vi "SampleClient.vi"() -> ()   [LabVIEW 2012]
doc: "A sample client that can be run on the computer or RIO"
panel:
  in  "Service call":bool
  out "Answer":string
  out "ms/iteration":dbl
  in  "Show Web":bool
  in  "LED":bool
  out "time":string
  out "Status":string
  in  "stop":bool
  # "Instructions:\n1. Run the VI\n2. Verify that you see the correct time.\n3. Press the LED button. You should see the LED reply change.\nIf you are targetting a myRIO, the LED should change as well.\n4. Debug by clicking Show Webpage.\n5. See what is being sent back and forth by clicking Show Webpage."
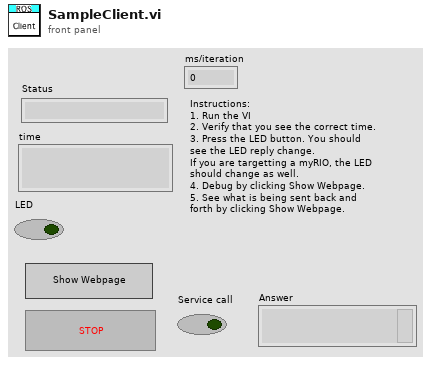
[diagram p1: front panel]
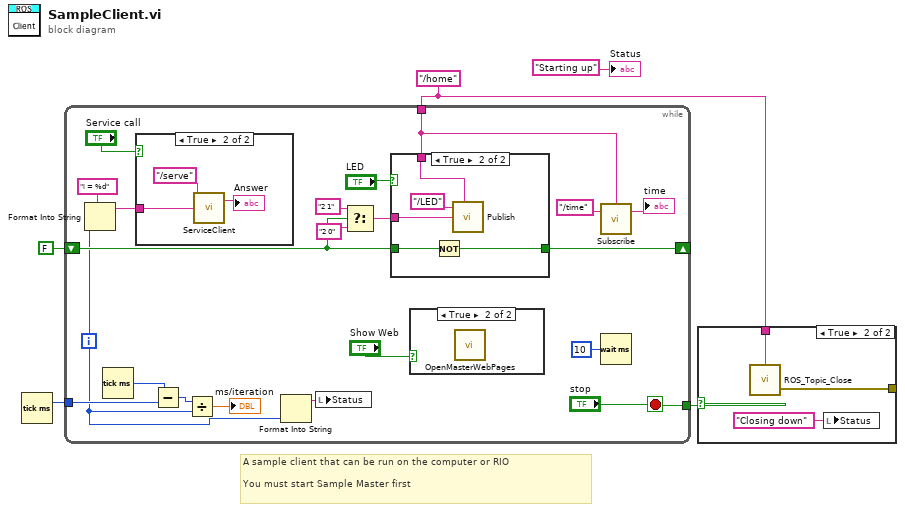
[diagram p0: block diagram]
diagram:
  w2 = "/home" ("Topic")
  # "A sample client that can be run on the computer or RIO\n\nYou must start Sample Master first"
  n1 = Tick Count (ms)() -> (millisecond timer value=w1:u32)
  n2 = while {
    tunnel: ["stop"] -> w3
    tunnel: w2 -> [w15]
    shift-right: [w21] -> _
    shift-left: FALSE -> [w20]
    tunnel: w1 -> [w12]
    i -> [w6]
    stop <- "stop" stop-if-true
    n3 = Format Into String(format string="i = %d" ("Msg in"), w6) -> (resulting string=w8:string)  [unwired: 2 in, 1 out]
    n4 = Tick Count (ms)() -> (millisecond timer value=w13:u32)
    n5 = case shown="True" "Service call" {
      tunnel: w8 -> [_ w28]
      frame False {
      }
      frame True {
        n6 = call <userlib>:"ServiceClient.vi"("Topic"="/serve", "Msg in"=w28) -> ("Reply"=→"Answer":string)  [unwired: 3 in, 1 out]
      }
    }
    n7 = Subtract(x=w13, y=w12) -> (x-y=w11:u32)
    n8 = Divide(x=w11, y=w6) -> (x/y=→"ms/iteration":dbl)
    n9 = Format Into String(w6) -> (resulting string=w25:string)  [unwired: 3 in, 1 out]
    n10 = local write "Status"(w25) -> ()
    n11 = Select(t="2 1" ("Status"), s=w20, f="2 0" ("Status")) -> (s? t:f=w22:string)
    n12 = case shown="True" "LED" {
      tunnel: w15 -> [_ w33]
      tunnel: w22 -> [_ w31]
      tunnel: [w30 w34] -> w21
      tunnel: w20 -> [w30 w35]
      frame False {
      }
      frame True {
        n13 = Not(x=w35) -> (.not. x?=w34:bool)
        n14 = call <userlib>:"Publish.vi"("Topic"="/LED", "node"=w33, "String"=w31) -> ()  [unwired: 4 in, 1 out]
      }
    }
    n15 = case shown="True" "Show Web" {
      frame False {
      }
      frame True {
        n16 = call <userlib>:"OpenMasterWebPages.vi"() -> ()  [unwired: 4 in]
      }
    }
    n17 = call <userlib>:"Subscribe.vi"("Topic"="/time", "node"=w15) -> ("Reply"=→"time":string)  [unwired: 1 in, 1 out]
    n18 = Wait (ms)(milliseconds to wait=u32 10) -> ()  [unwired: 1 out]
  }
  n19 = case shown="True" w3 {
    tunnel: w2 -> [_ w37]
    tunnel: [_ w36] -> _
    frame False {
    }
    frame True {
      n20 = call <userlib>:"ROS_Topic_Close.vi"("node"=w37) -> ("error out"=w36:errorcluster)  [unwired: 3 in]
      n21 = local write "Status"("Closing down" ("Status")) -> ()
    }
  }
  "Status" <- "Starting up" ("Status")
